vi "PC_CTRL.vi"() -> ()   [LabVIEW 2014]
panel:
  out "Start time":cluster{timestamp[], i32[]}(graph)
  out "Temp":cluster{timestamp[], i32[]}(graph)
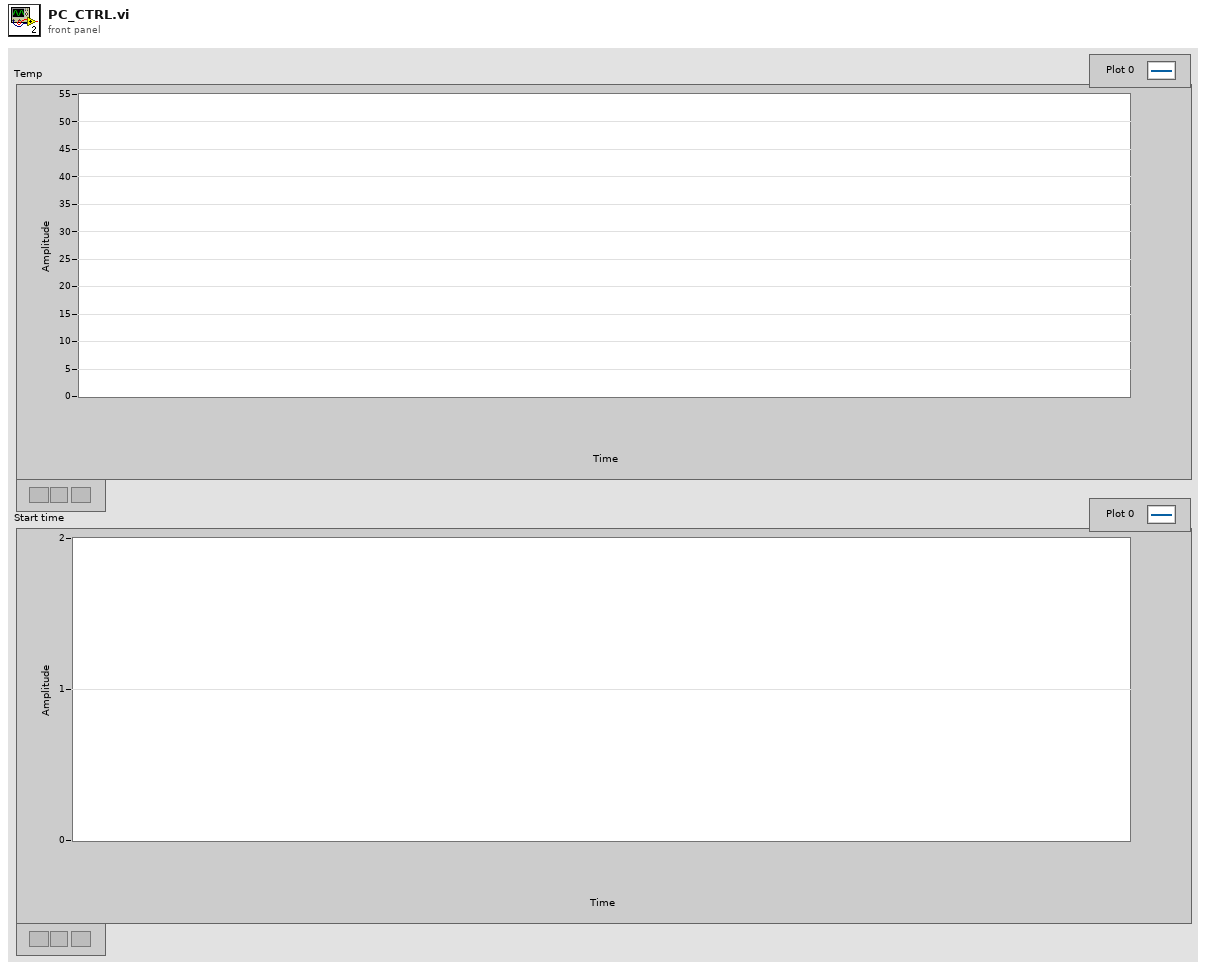
[diagram p1: front panel]
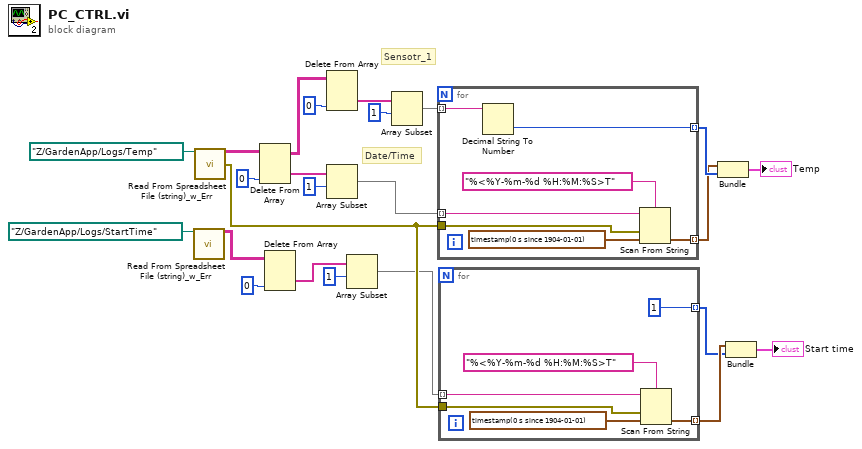
[diagram p0: block diagram]
diagram:
  # "Sensotr_1"
  # "Date/Time"
  n1 = call "Read From Spreadsheet File (string)_w_Err.vi"("file path (dialog if empty)"=path "Z:/GardenApp/Logs/StartTime") -> ("all rows"=w9:string[][])  [unwired: 9 in, 5 out]
  n2 = call "Read From Spreadsheet File (string)_w_Err.vi"("file path (dialog if empty)"=path "Z:/GardenApp/Logs/Temp") -> ("all rows"=w23:string[][], "error out"=w5:errorcluster)  [unwired: 9 in, 4 out]
  n3 = Delete From Array(array=w23, index (col)=0 ("disabled index (col)")) -> (deleted portion=w21:string[], array with subset deleted=w19:string[][])  [unwired: 2 in]
  n4 = Delete From Array(array=w9, index (col)=0 ("disabled index (col)")) -> (deleted portion=w6:string[])  [unwired: 2 in, 1 out]
  n5 = Delete From Array(array=w19, index (col)=0 ("disabled index (col)")) -> (deleted portion=w16:string[])  [unwired: 2 in, 1 out]
  n6 = Array Subset(array=w21, index=1) -> (w15:string[])  [unwired: 1 in]
  n7 = Array Subset(array=w6, index=1) -> (w1:string[])  [unwired: 1 in]
  n8 = Array Subset(array=w16, index=1) -> (w14:string[])  [unwired: 1 in]
  n9 = for {
    tunnel: w15 -> [w29] mode=indexing
    tunnel: w14 -> [w31] mode=indexing
    tunnel: [w30] -> w12 mode=indexing
    tunnel: [w27] -> w11 mode=indexing
    tunnel: w5 -> [w25]
    n10 = Decimal String To Number(string=w31) -> (number=w30:i32)  [unwired: 2 in, 1 out]
    n11 = Scan From String(format string="%<%Y-%m-%d %H:%M:%S>T", input string=w29, error in=w25, default 1=timestamp(0 s since 1904-01-01)) -> (output 1=w27:timestamp)  [unwired: 1 in, 3 out]
  }
  n12 = for {
    tunnel: w1 -> [w32] mode=indexing
    tunnel: [w36] -> w4 mode=indexing
    tunnel: w5 -> [w34]
    tunnel: [1] -> w3 mode=indexing
    n13 = Scan From String(format string="%<%Y-%m-%d %H:%M:%S>T", input string=w32, error in=w34, default 1=timestamp(0 s since 1904-01-01)) -> (output 1=w36:timestamp)  [unwired: 1 in, 3 out]
  }
  n14 = Bundle(w11, w12) -> (→"Temp":cluster{timestamp[], i32[]})  [unwired: 1 in]
  n15 = Bundle(w4, w3) -> (→"Start time":cluster{timestamp[], i32[]})  [unwired: 1 in]
